vi "Actor Receive Core.vi"(10 "Msg in":refnum<class "Msg Strategy.lvclass">, 11 "Msging Self Actor State in":refnum<class "Msging Self Actor State.lvclass">) -> (2 "Msg out":refnum<class "Msg Strategy.lvclass">)   [LabVIEW 2021, in "LVCAM.lvlib" / "Msging Self Actor State.lvclass"]
uses:
  Msging Self Actor State.lvclass
  Msg Strategy/Msg Strategy.lvclass
  Msging Self Actor State.lvclass/Msging Self Actor State.ctl
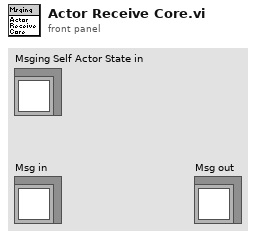
[diagram p1: front panel]
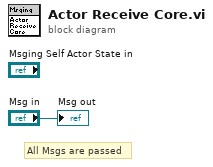
[diagram p0: block diagram]
diagram:
  # "All Msgs are passed"
  "Msg out" <- "Msg in"
